vi "Stop.vi"(8 "error in (no error)":errorcluster, 11 "1553 Component in":refnum<class "1553 Component.lvclass">) -> (0 "error out":errorcluster, 3 "1553 Component out":refnum<class "1553 Component.lvclass">)   [LabVIEW 2020, in "BCI-1553 API.lvlib" / "1553 Component.lvclass"]
doc: "Stops the operation of a component that has already been started."
uses:
  1553 Component.lvclass
  1553 Component.lvclass/1553 Component.ctl
  1553 SubComponent/1553 SubComponent.lvclass
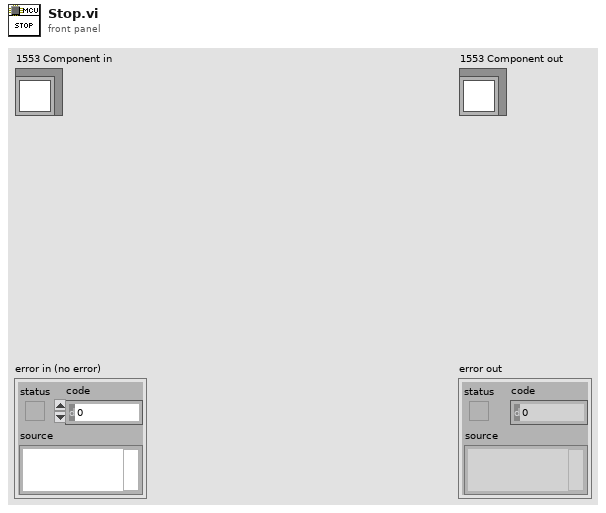
[diagram p1: front panel]
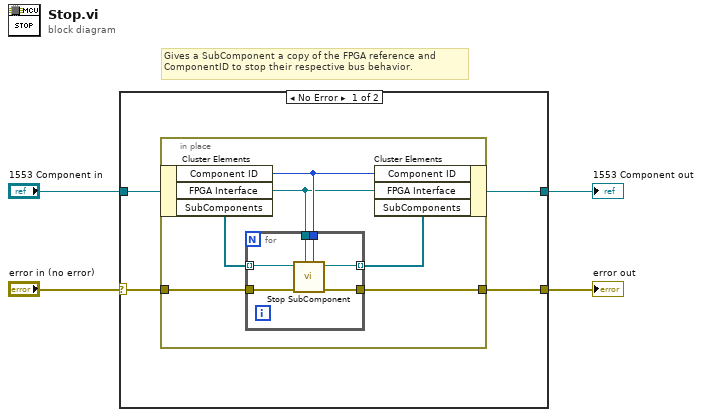
[diagram p0: block diagram]
diagram:
  # "Gives a SubComponent a copy of the FPGA reference and\nComponentID to stop their respective bus behavior."
  n1 = case shown="No Error" "error in (no error)" {
    selector: "error in (no error)" -> [w8 w22]
    tunnel: [w7 w22] -> w1
    tunnel: [w5 w21] -> w2
    tunnel: "1553 Component in" -> [w6 w21]
    frame No Error {
      n2 = in-place {
        in-place-border: w8 -> [w12]
        in-place-border: [w11] -> w7
        n3 = in-place-cluster #1(w6) -> ("Component ID"=w10:u8, "FPGA Interface"=w9:refnum<class "FPGA Interface.lvclass">, "SubComponents"=w14:refnum<class "1553 SubComponent.lvclass">[])
        n4 = for {
          tunnel: w14 -> [w20] mode=indexing
          tunnel: [w15] -> w13 mode=indexing
          tunnel: w12 -> [w18]
          tunnel: [w19] -> w11
          tunnel: w9 -> [w17]
          tunnel: w10 -> [w16]
          n5 = call-dynamic "Stop SubComponent.vi"("Component ID"=w16, "FPGA Interface"=w17, "error in (no error)"=w18, "1553 SubComponent in"=w20) -> ("error out"=w19:errorcluster, "1553 SubComponent out"=w15:refnum<class "1553 SubComponent.lvclass">)  [unwired: 6 in]
        }
        n6 = in-place-cluster #1("Component ID"=w10, "FPGA Interface"=w9, "SubComponents"=w13) -> (w5:refnum<class "1553 Component.lvclass">)
      }
    }
    frame Error {
    }
  }
  "error out" <- w1
  "1553 Component out" <- w2
